vi "Set Manual Mode.vi"(6 "Heater Range (0: Off)":u16(ring) items=["Off", "Low (0.5W)", "Med (5W)", "High (50W)"], 8 "error in (no error)":errorcluster, 9 "Power":dbl, 10 "Manual Mode":bool, 11 "Lakeshore 325 in":refnum<class "Lakeshore 325.lvclass">) -> (0 "error out":errorcluster, 3 "Lakeshore 325 out":refnum<class "Lakeshore 325.lvclass">)   [LabVIEW 2022 SP3, in "Lakeshore 325.lvclass"]
uses:
  Lakeshore 325.lvclass
  Lakeshore 325.lvclass/Lakeshore 325.ctl
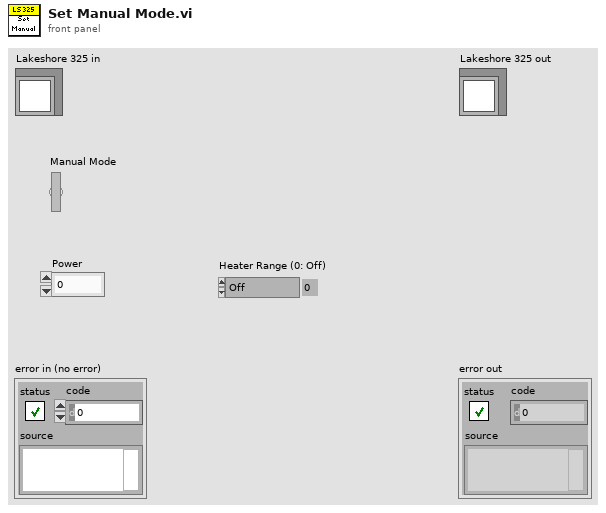
[diagram p1: front panel]
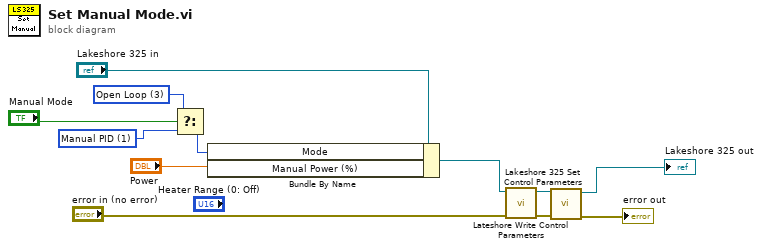
[diagram p0: block diagram]
diagram:
  w8 = u16 1 items=["Manual PID"=1, "Zone"=2, "Open Loop"=3, "AutoTune PID"=4, "AutoTune PI"=5, "AutoTune P"=6] ("Mode (1:Manual PID)")
  w9 = u16 3 items=["Manual PID"=1, "Zone"=2, "Open Loop"=3, "AutoTune PID"=4, "AutoTune PI"=5, "AutoTune P"=6] ("Mode (1:Manual PID)")
  n1 = Select(t=w9, s="Manual Mode", f=w8) -> (s? t:f=w7:u16)
  n2 = Bundle By Name(cluster="Lakeshore 325 in", "Mode"=w7, "Manual Power (%)"="Power") -> (w4:refnum<class "Lakeshore 325.lvclass">)
  n3 = call "Lateshore Write Control Parameters.vi"("error in (no error)"="error in (no error)", "Lakeshore 325 in"=w4) -> ("error out"=w1:errorcluster, "Lakeshore 325 out"=w3:refnum<class "Lakeshore 325.lvclass">)  [unwired: 8 in]
  n4 = call "Lakeshore 325 Set Control Parameters.vi"("error in (no error)"=w1, "Lakeshore 325 in"=w3) -> ("error out"=→"error out":errorcluster, "Lakeshore 325 out"=→"Lakeshore 325 out":refnum<class "Lakeshore 325.lvclass">)  [unwired: 8 in]
